vi "rqcBob Get Detector State (1 SPD).vi"(0 "SPD1 signal":bool, 1 "enable write":bool, 9 "window":bool, 11 "clock in":bool, 12 "DAC level":u8) -> (4 "SPD state":u16, 10 "write to fifo":bool)   [LabVIEW 2016]
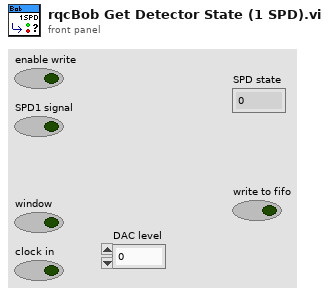
[diagram p1: front panel]
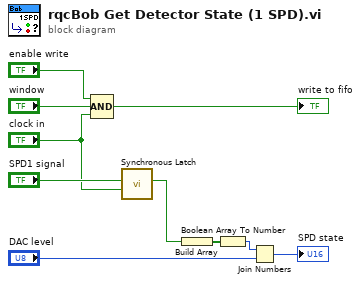
[diagram p0: block diagram]
diagram:
  n1 = Compound Arithmetic op=AND("enable write", "window", "clock in") -> (→"write to fifo":bool)
  n2 = call <vilib>:"Synchronous Latch.vi"("clear"="clock in", "set"="SPD1 signal") -> ("out"=w4:bool)  [unwired: 9 in]
  n3 = Build Array(w4) -> (w3:bool[])
  n4 = Boolean Array To Number(Boolean array=w3) -> (number=w2:u8)
  n5 = Join Numbers(hi=w2, lo="DAC level") -> ((hi.lo)=→"SPD state":u16)
